vi "Main.vi"() -> ()   [LabVIEW 2019]
uses:
  <vilib>/Platform/TimedLoop/XDataNode/timing_clust.ctl
  <vilib>/Platform/TimedLoop/XDataNode/nitl_modes.ctl
  <vilib>/Platform/TimedLoop/XDataNode/wakeup.ctl
  <vilib>/Analysis/3filter.llb/Filter Passband Type.ctl
  init_var.ctl
  <vilib>/addons/control/pid/pid.llb/PID (DBL).vi
  <vilib>/Platform/TimedLoop/XDataNode/XDataNode.xnode
  KNRm_ReMi_OS6_436Motor.lvlibp
  <vilib>/Platform/TimedLoop/XDataNode/XDNodeRunTimeDep.lvlib
  <vilib>/addons/control/pid/NI_PID_pid.lvlib
  <vilib>/ptbypt/NI_PtbyPt.lvlib
  <vilib>/Analysis/NI_AALBase.lvlib
panel:
  in  "步進馬達程式":bool=TRUE
  in  "模擬程式":bool=TRUE
  out "結構是否合理":bool=TRUE
  out "IR":dbl=-23.857993553151026 format="%0.2f"
  out "Stepdeg":dbl=0.19285714285714284 format="%#_2g"
  out "模擬圖":cluster{dbl[], dbl[]}[](graph)=[{[62.44507934888324, 68.04507807993414, 67.49670850165072, 50.0, 62.44507934888324], [50.0, 49.99623008910044, 62.78447824143207, 62.44507934888324, 50.0]}, {array[360 elements], array[360 elements]}, {[33.0, 67.0], [62.11531554372036, 62.774843154046124]}, {[38.25, 38.25], [70.0, 50.0]}]
  in  "Target(+/-)25":dbl(slide)=-25.0 min=25.0 step=1.0 scale=25.0..-25.0 scale format="%#_3g"
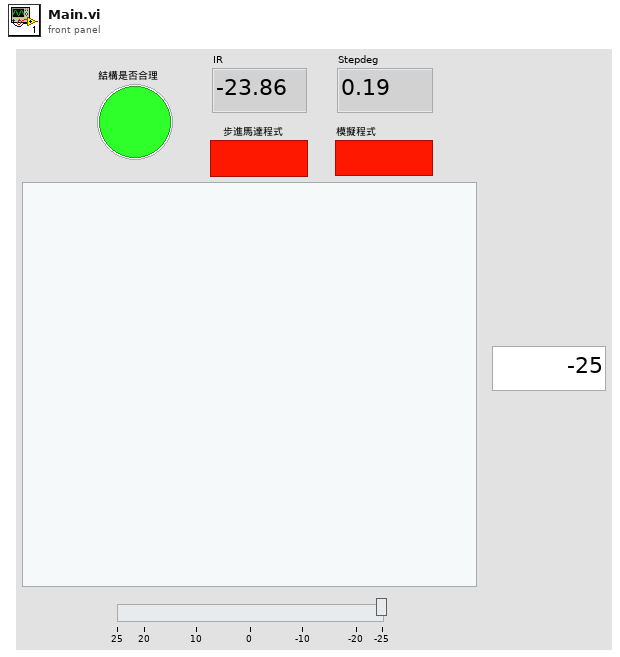
[diagram p1: front panel]
types:
  T1 = typedef "XDNodeRunTimeDep.lvlib/timing_clust.ctl" = cluster{"Expected End [f-1]":u64, "Actual End [f-1]":u64, "Finished Late? [f-1]":bool, "Expected End [i-1]":u64, "Actual End [i-1]":u64, "Finished Late? [i-1]":bool, "Expected Start [i]":u64, "Actual Start [i]":u64, "Expected Start [f]":u64, "Actual Start [f]":u64, "Source Name":string, "Structure Name":string, "Period":i64, "Deadline":i64, "Offset":i64, "Start":i64, "Priority":i32, "Timeout":i32, "Mode":T2, "Wakeup Reason":T3, "Error":errorcluster, "Source Type":string, "Secondary Source Type":string, "Global End Time":u64, "Global Start Time":u64, "Frame Duration":u64, "Iteration Duration":u64, "Assigned CPU":i32, "I/O Scan Engine Mode":u32}
  T2 = typedef "XDNodeRunTimeDep.lvlib/nitl_modes.ctl" = enum32{"No Change", "Process missed periods, maintain original phase", "Discard missed periods, maintain original phase", "Process missed periods, ignore original phase", "Discard missed periods, ignore original phase"}
  T3 = typedef "XDNodeRunTimeDep.lvlib/wakeup.ctl" = enum32{"Normal", "Aborted", "Asynchronous wakeup", "Timing source error", "Timed loop error", "Timeout"}
  T4 = typedef "init_var.ctl" = cluster{"L1":dbl, "L2":dbl, "L3":dbl, "L4":dbl, "θ1":dbl, "θ2":dbl}
  T5 = cluster{"proportional gain (Kc)":dbl, "integral time (Ti, min)":dbl, "derivative time (Td, min)":dbl}
  T6 = typedef "NI_AALBase.lvlib/Filter Passband Type.ctl" = enum32{"Lowpass", "Highpass", "Bandpass", "Bandstop"}
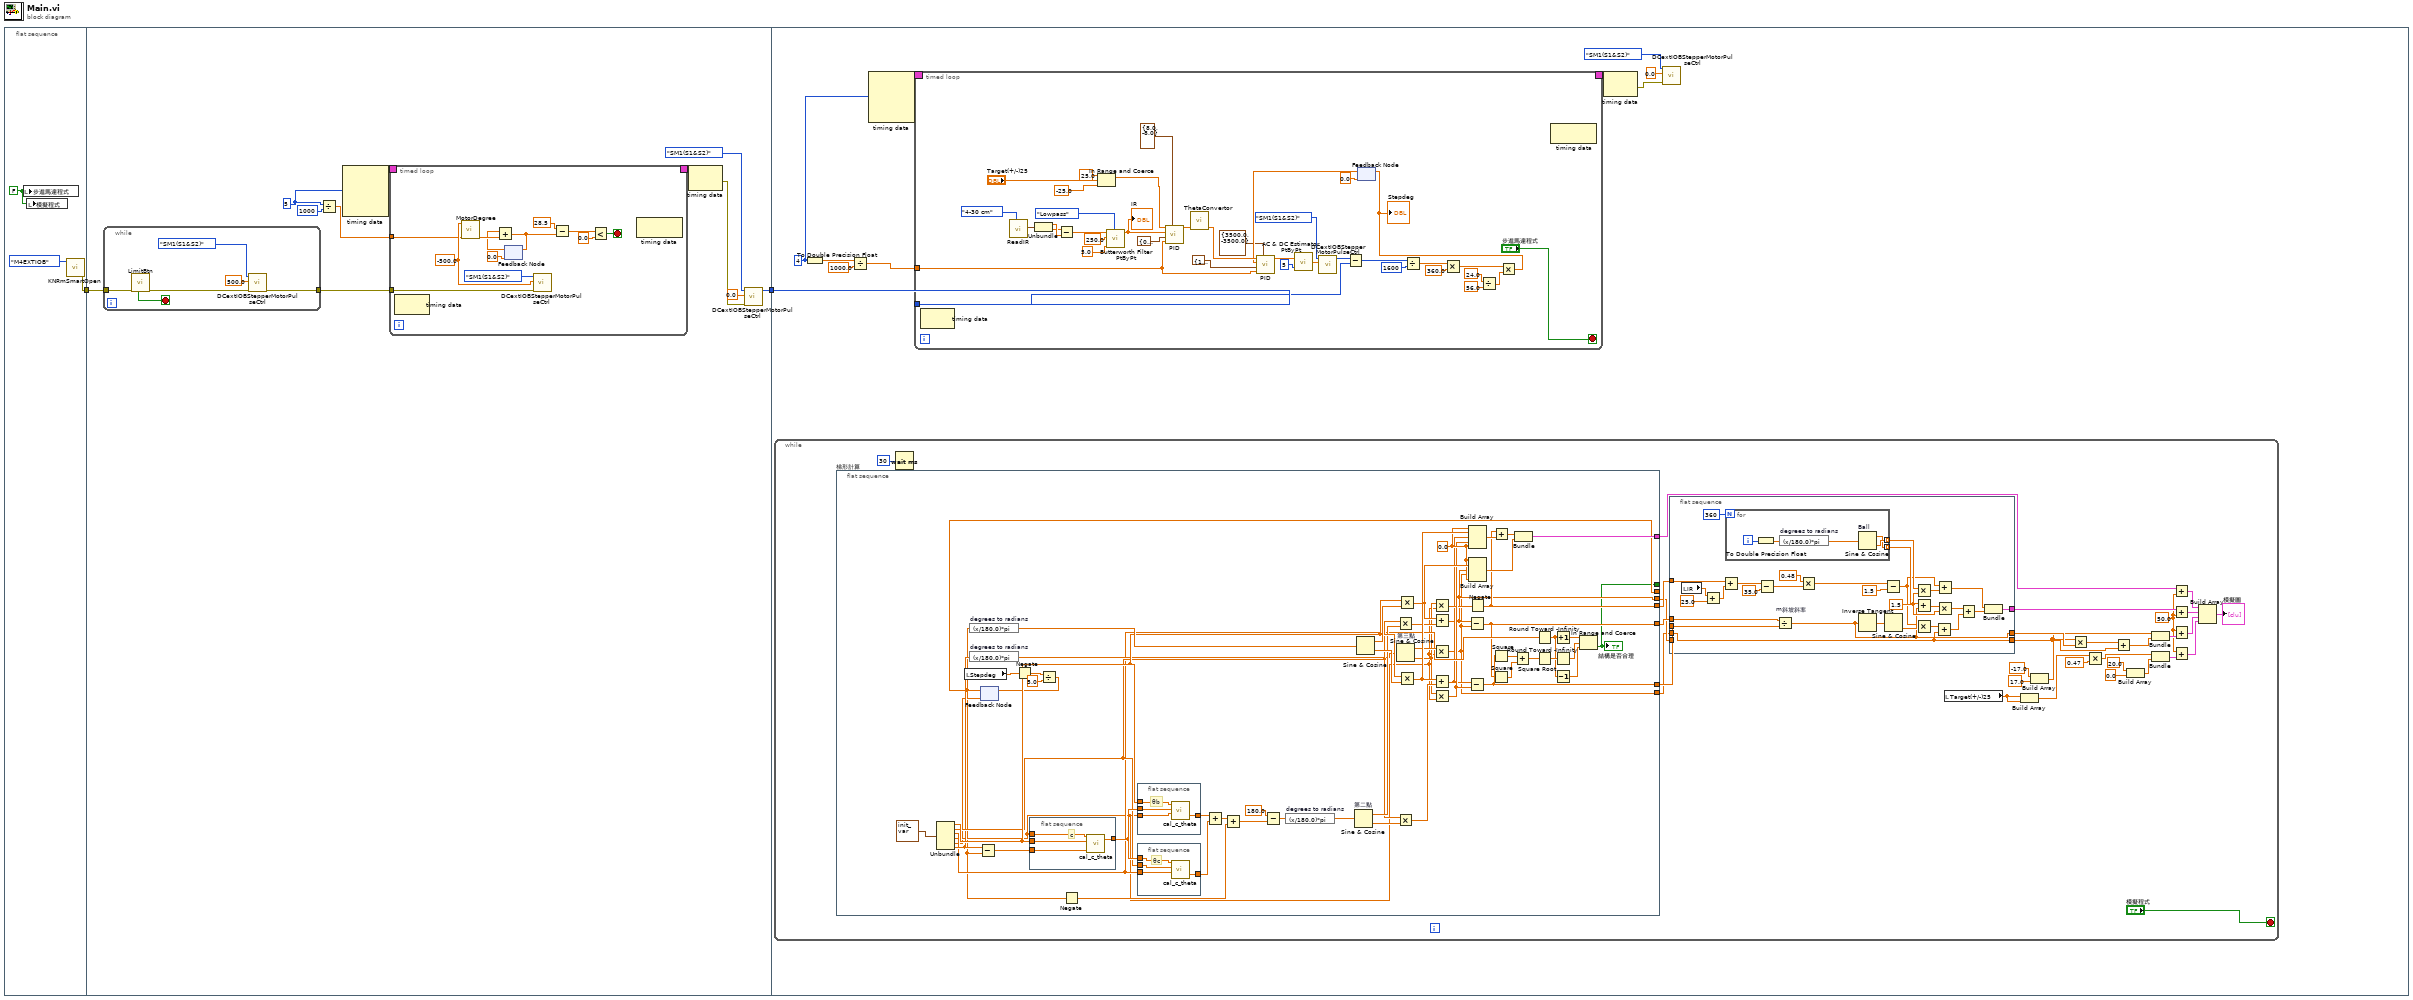
[diagram p0: block diagram]
diagram:
  n1 = flat-sequence {
    tunnel: [w3] -> w1
    tunnel: [w6] -> w2
    tunnel: w1 -> [w15]
    tunnel: w2 -> [w42]
    frame #0 {
      w5 = FALSE ("步進馬達程式")
      n2 = local write "步進馬達程式"(w5) -> ()
      n3 = local write "模擬程式"(w5) -> ()
      n4 = call "KNRmSmartOpen.vi"("INI FPGA MODE"=enum16{"Original", "M4EXTIOB"}."M4EXTIOB") -> ("error out"=w3:errorcluster)  [unwired: 7 in, 3 out]
    }
    frame #1 {
      w12 = i64 5 ("Period")
      n5 = while {
        tunnel: [w40] -> w16
        tunnel: w15 -> [w36]
        stop <- w38 stop-if-true
        n6 = call "LimitBtn.vi"("error in"=w36) -> ("error out"=w37:errorcluster, "LimitBtn"=w38:bool)  [unwired: 9 in]
        n7 = call "DCextIOBStepperMotorPulseCtrl.vi"("error in"=w37, "PulseRate&Dir P/S"=500.0 ("Pulse(Hz) and direction"), "Port"=enum16{"SM1(S1&S2)", "SM2(S3&S4)", "SM3(S5&S6)"}."SM1(S1&S2)") -> ("error out"=w40:errorcluster)  [unwired: 7 in, 1 out]
      }
      n8 = Divide(x=w12, y=i64 1000) -> (x/y=w10:dbl)
      n9 = node-c288(w12) -> (w14:T1)  [unwired: 3 in]
      n10 = timed-loop {
        tunnel: w16 -> [w28]
        timing: w14 -> [_]
        timing-out: [_] -> w13
        tunnel: w10 -> [w21]
        stop <- w24 stop-if-true
        w22 = -500.0 ("Pulse(Hz) and direction")
        n11 = node-c288() -> ()  [unwired: 1 in, 1 out]
        n12 = call "MotorDegree.vi"("Looptime"=w21, "Pulse(Hz) and direction"=w22) -> ("MotorVel"=w20:dbl)  [unwired: 9 in]
        n13 = feedback #1(0.0) -> (w19:dbl)
        n14 = Add(x=w19, y=w20) -> (x+y=w17:dbl)
        n15 = feedback-in #1(w17) -> ()
        n16 = call "DCextIOBStepperMotorPulseCtrl.vi"("error in"=w28, "PulseRate&Dir P/S"=w22, "Port"=enum16{"SM1(S1&S2)", "SM2(S3&S4)", "SM3(S5&S6)"}."SM1(S1&S2)") -> ()  [unwired: 7 in, 2 out]
        n17 = Subtract(x=28.5, y=w17) -> (x-y=w26:dbl)
        n18 = Less?(x=w26, y=0.0) -> (x < y?=w24:bool)
        n19 = node-c288() -> ()  [unwired: 1 in, 1 out]
      }
      n20 = node-c288(w13) -> (w7:errorcluster)
      n21 = call "DCextIOBStepperMotorPulseCtrl.vi"("error in"=w7, "PulseRate&Dir P/S"=0.0, "Port"=enum16{"SM1(S1&S2)", "SM2(S3&S4)", "SM3(S5&S6)"}."SM1(S1&S2)") -> ("PulseCounter+/-"=w6:i32)  [unwired: 7 in, 1 out]
    }
    frame #2 {
      w47 = i64 4 ("Period")
      n22 = while {
        stop <- "模擬程式" stop-if-true
        w56 = 50.0 ("θ1")
        n23 = flat-sequence "梯形計算" {
          tunnel: [w141] -> w77
          tunnel: [w140] -> w81
          tunnel: [w139] -> w80
          tunnel: [w126] -> _
          tunnel: [w120] -> _
          tunnel: [w128] -> w75
          tunnel: [w122] -> w68
          tunnel: [w121] -> w67
          frame #0 {
            w151 = 0.0 ("element")
            n24 = Unbundle(T4 {"L1"=5.6, "L2"=12.8, "L3"=17.5, "L4"=17.6, "θ1"=0.0, "θ2"=135.0} ("初始設定")) -> ("L1"=w162:dbl, "L2"=w159:dbl, "L3"=w142:dbl, "L4"=w131:dbl, "θ1"=w127:dbl, "θ2"=w150:dbl)
            n25 = local read "Stepdeg"() -> (w119:dbl)
            n26 = expression code="(x/180.0)*pi" "degrees to radians"(w150) -> (w149:dbl)
            n27 = feedback #2(w127) -> (w126:dbl)
            n28 = expression code="(x/180.0)*pi" "degrees to radians"(w126) -> (w167:dbl)
            n29 = Subtract(x=w150, y=w126) -> (x-y=w165:dbl)
            n30 = Negate(x=w119) -> (-x=w118:dbl)
            n31 = flat-sequence {
              tunnel: [w184] -> w164
              tunnel: w165 -> [w183]
              tunnel: w131 -> [w182]
              tunnel: w162 -> [w181]
              frame #0 {
                # "c"
                n32 = call "cal_c_theta.vi"("θ"=w183, "b"=w181, "a"=w182) -> ("c"=w184:dbl)  [unwired: 1 in, 1 out]
              }
            }
            n33 = Divide(x=w118, y=5.0 ("x")) -> (x/y=w125:dbl)
            n34 = feedback-in #2(w125) -> ()
            n35 = Negate(x=w126) -> (-x=w147:dbl)
            n36 = flat-sequence {
              tunnel: [w180] -> w172
              tunnel: w162 -> [w179]
              tunnel: w164 -> [w178]
              tunnel: w131 -> [w177]
              frame #0 {
                # "θb"
                n37 = call "cal_c_theta.vi"("c"=w177, "b"=w178, "a"=w179) -> ("theta"=w180:dbl)  [unwired: 1 in, 1 out]
              }
            }
            n38 = flat-sequence {
              tunnel: [w173] -> w171
              tunnel: w164 -> [w176]
              tunnel: w159 -> [w175]
              tunnel: w142 -> [w174]
              frame #0 {
                # "θc"
                n39 = call "cal_c_theta.vi"("c"=w174, "b"=w175, "a"=w176) -> ("theta"=w173:dbl)  [unwired: 1 in, 1 out]
              }
            }
            n40 = Add(x=w172, y=w171) -> (x+y=w168:dbl)
            n41 = Add(x=w168, y=w147) -> (x+y=w169:dbl)
            n42 = Subtract(x=180.0 ("θ1"), y=w169) -> (x-y=w152:dbl)
            n43 = expression code="(x/180.0)*pi" "degrees to radians"(w152) -> (w166:dbl)
            n44 = Sine & Cosine "第二點"(0:w166) -> (1:w160:dbl, 2:w158:dbl)
            n45 = Sine & Cosine(0:w167) -> (1:w163:dbl, 2:w161:dbl)
            n46 = Multiply(x=w159, y=w160) -> (x*y=w154:dbl)
            n47 = Sine & Cosine "第三點"(0:w149) -> (1:w148:dbl, 2:w132:dbl)
            n48 = Multiply(x=w159, y=w158) -> (x*y=w153:dbl)
            n49 = Multiply(x=w162, y=w163) -> (x*y=w155:dbl)
            n50 = Multiply(x=w162, y=w161) -> (x*y=w156:dbl)
            n51 = Multiply(x=w132, y=w131) -> (x*y=w129:dbl)
            n52 = Add(x=w155, y=w154) -> (x+y=w122:dbl)
            n53 = Multiply(x=w148, y=w131) -> (x*y=w121:dbl)
            n54 = Add(x=w156, y=w153) -> (x+y=w123:dbl)
            n55 = Multiply(x=w132, y=w131) -> (x*y=w134:dbl)
            n56 = Subtract(x=w122, y=w121) -> (x-y=w139:dbl)
            n57 = Subtract(x=w123, y=w134) -> (x-y=w140:dbl)
            n58 = Build Array(w151, w156, w123, w134, w151) -> (w133:dbl[])
            n59 = Build Array(w151, w155, w122, w121, w151) -> (w157:dbl[])
            n60 = Negate(x=w129) -> (-x=w128:dbl)
            n61 = Square(x=w140) -> (x^2=w146:dbl)
            n62 = Square(x=w139) -> (x^2=w145:dbl)
            n63 = Add(x=w128, y=w133) -> (x+y=w130:dbl[])
            n64 = Add(x=w146, y=w145) -> (x+y=w144:dbl)
            n65 = Bundle(w130, w157) -> (w141:cluster{dbl[], dbl[]})  [unwired: 1 in]
            n66 = Round Toward -Infinity(1:w142) -> (0:w136:dbl)
            n67 = Square Root(x=w144) -> (sqrt(x)=w143:dbl)
            n68 = Increment(x=w136) -> (x+1=w137:dbl)
            n69 = Round Toward -Infinity(1:w143) -> (0:w138:dbl)
            n70 = Decrement(x=w136) -> (x-1=w135:dbl)
            n71 = In Range and Coerce(upper limit=w137, x=w138, lower limit=w135) -> (In Range?=w120:bool)  [unwired: 1 out]
            "結構是否合理" <- w120
          }
        }
        n72 = Wait (ms)(milliseconds to wait=u32 30) -> ()  [unwired: 1 out]
        n73 = flat-sequence {
          tunnel: w81 -> [w110]
          tunnel: w80 -> [w109]
          tunnel: [w108] -> w79
          tunnel: w75 -> [w96]
          tunnel: [w92] -> w71
          tunnel: w68 -> [_]
          tunnel: w67 -> [w88]
          tunnel: [w88] -> w66
          frame #0 {
            w106 = 1.5 ("θ1")
            n74 = local read "IR"() -> (w85:dbl)
            n75 = Add(x=w85, y=25.0) -> (x+y=w83:dbl)
            n76 = Add(x=w96, y=w83) -> (x+y=w97:dbl)
            n77 = for {
              N: 360 -> [_]
              tunnel: [w113] -> w100 mode=indexing
              tunnel: [w112] -> w105 mode=indexing
              i -> [w115]
              n78 = To Double Precision Float(number=w115) -> (double precision float=w114:dbl)
              n79 = expression code="(x/180.0)*pi" "degrees to radians"(w114) -> (w116:dbl)
              n80 = Sine & Cosine "Ball"(0:w116) -> (1:w112:dbl, 2:w113:dbl)
            }
            n81 = Subtract(x=w97, y=35.0) -> (x-y=w98:dbl)
            n82 = Divide "m斜坡斜率"(x=w109, y=w110) -> (x/y=w92:dbl)
            n83 = Multiply(x=0.48, y=w98) -> (x*y=w93:dbl)
            n84 = Inverse Tangent(1:w92) -> (0:w107:dbl)
            n85 = Subtract(x=w93, y=1.5 ("球位置補償")) -> (x-y=w91:dbl)
            n86 = Sine & Cosine(0:w107) -> (2:w99:dbl)  [unwired: 1 out]
            n87 = Multiply(x=w100, y=w106) -> (x*y=w101:dbl[])
            n88 = Add(x=w105, y=w99) -> (x+y=w103:dbl[])
            n89 = Multiply(x=w91, y=w92) -> (x*y=w90:dbl)
            n90 = Add(x=w90, y=w88) -> (x+y=w89:dbl)
            n91 = Add(x=w91, y=w101) -> (x+y=w94:dbl[])
            n92 = Multiply(x=w103, y=w106) -> (x*y=w104:dbl[])
            n93 = Add(x=w104, y=w89) -> (x+y=w102:dbl[])
            n94 = Bundle(w94, w102) -> (w108:cluster{dbl[], dbl[]})  [unwired: 1 in]
          }
        }
        n95 = local read "Target(+/-)25"() -> (w62:dbl)
        n96 = Build Array(w62, w62) -> (w54:dbl[])
        n97 = Build Array(-17.0 ("element"), 17.0 ("element")) -> (w61:dbl[])
        n98 = Multiply(x=w61, y=w71) -> (x*y=w70:dbl[])
        n99 = Multiply(x=w54, y=0.47 ("element")) -> (x*y=w53:dbl[])
        n100 = Add(x=w70, y=w66) -> (x+y=w69:dbl[])
        n101 = Build Array(20.0 ("element"), 0.0 ("element")) -> (w59:dbl[])
        n102 = Bundle(w61, w69) -> (w74:cluster{dbl[], dbl[]})  [unwired: 1 in]
        n103 = Bundle(w53, w59) -> (w57:cluster{dbl[], dbl[]})  [unwired: 1 in]
        n104 = Add(x=w77, y=w56) -> (x+y=w76:cluster{dbl[], dbl[]})
        n105 = Add(x=w79, y=w56) -> (x+y=w82:cluster{dbl[], dbl[]})
        n106 = Add(x=w56, y=w74) -> (x+y=w64:cluster{dbl[], dbl[]})
        n107 = Add(x=w56, y=w57) -> (x+y=w55:cluster{dbl[], dbl[]})
        n108 = Build Array(w76, w82, w64, w55) -> (→"模擬圖":cluster{dbl[], dbl[]}[])
      }
      n109 = To Double Precision Float(number=w47) -> (double precision float=w49:dbl)
      n110 = Divide(x=w49, y=1000.0) -> (x/y=w46:dbl)
      n111 = node-c288(w47) -> (w51:T1)  [unwired: 3 in]
      n112 = timed-loop {
        timing: w51 -> [_]
        timing-out: [_] -> w50
        tunnel: w46 -> [w203]
        tunnel: w42 -> [w191]
        stop <- "步進馬達程式" stop-if-true
        n113 = node-c288() -> ()  [unwired: 1 in, 1 out]
        n114 = call "ReadIR.vi"("type"=enum16{"10-80 cm", "4-30 cm"}."4-30 cm") -> ("Distance (cm)"=w197:cluster{"IR1":dbl, "IR2":dbl})  [unwired: 8 in, 2 out]
        n115 = Unbundle(w197) -> ("IR1"=w199:dbl, "IR2"=w198:dbl)
        n116 = Subtract(x=w198, y=w199) -> (x-y=w193:dbl)
        n117 = In Range and Coerce(upper limit=25.0, x="Target(+/-)25", lower limit=-25.0) -> (coerced(x)=w187:dbl)  [unwired: 1 out]
        n118 = call <vilib>:"Butterworth Filter PtByPt.vi"("filter type"=Filter_Passband_Type."Lowpass", "low cutoff freq: fl"=5.0, "sampling freq: fs"=250.0, "x"=w193) -> ("Filtered x"=w192:dbl)  [unwired: 5 in, 1 out]
        "IR" <- w192
        n119 = call-poly <vilib>:"PID.vi"("output range"=cluster{"output high":dbl, "output low":dbl} {"output high"=8.0, "output low"=-8.0}, "dt (s)"=w203, "PID gains"=T5 {"proportional gain (Kc)"=0.29999999999999993, "integral time (Ti, min)"=0.03, "derivative time (Td, min)"=0.012999999999999998} ("PosPID"), "process variable"=w192, "setpoint"=w187) -> ("output"=w200:dbl)  [unwired: 5 in, 1 out]
        n120 = call "ThetaConvertor.vi"("Theta2IN"=w200) -> ("Theta1OUT"=w220:dbl)  [unwired: 9 in, 1 out]
        n121 = feedback #3(0.0) -> (w216:dbl)
        n122 = call-poly <vilib>:"PID.vi"("output range"=cluster{"output high":dbl, "output low":dbl} {"output high"=3500.0, "output low"=-3500.0}, "dt (s)"=w203, "PID gains"=T5 {"proportional gain (Kc)"=100.0, "integral time (Ti, min)"=0.0, "derivative time (Td, min)"=0.0} ("StepperPID"), "process variable"=w216, "setpoint"=w220) -> ("output"=w206:dbl)  [unwired: 5 in, 1 out]
        n123 = call <vilib>:"AC & DC Estimator PtByPt.vi"("signal"=w206, "sample length"=5) -> ("DC estimate (V)"=w204:dbl)  [unwired: 1 in, 2 out]
        n124 = call "DCextIOBStepperMotorPulseCtrl.vi"("PulseRate&Dir P/S"=w204, "Port"=enum16{"SM1(S1&S2)", "SM2(S3&S4)", "SM3(S5&S6)"}."SM1(S1&S2)") -> ("PulseCounter+/-"=w208:i32)  [unwired: 8 in, 1 out]
        n125 = Subtract(x=w208, y=w191) -> (x-y=w207:i32)
        n126 = Divide(x=w207, y=1600) -> (x/y=w218:dbl)
        n127 = Multiply(x=w218, y=360.0) -> (x*y=w212:dbl)
        n128 = Divide(x=24.0, y=56.0) -> (x/y=w211:dbl)
        n129 = Multiply(x=w212, y=w211) -> (x*y=w210:dbl)
        "Stepdeg" <- w210
        n130 = feedback-in #3(w210) -> ()
        n131 = node-c288() -> ()  [unwired: 1 in, 1 out]
      }
      n132 = node-c288(w50) -> (w43:errorcluster)
      n133 = call "DCextIOBStepperMotorPulseCtrl.vi"("error in"=w43, "PulseRate&Dir P/S"=0.0 ("Pulse(Hz) and direction"), "Port"=enum16{"SM1(S1&S2)", "SM2(S3&S4)", "SM3(S5&S6)"}."SM1(S1&S2)") -> ()  [unwired: 7 in, 2 out]
    }
  }
